vi "(17) part 2 que.vi"() -> ()   [LabVIEW 2025]
panel:
  out "Numeric 2":dbl
  in  "Numeric":dbl
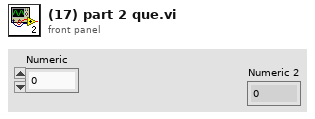
[diagram p1: front panel]
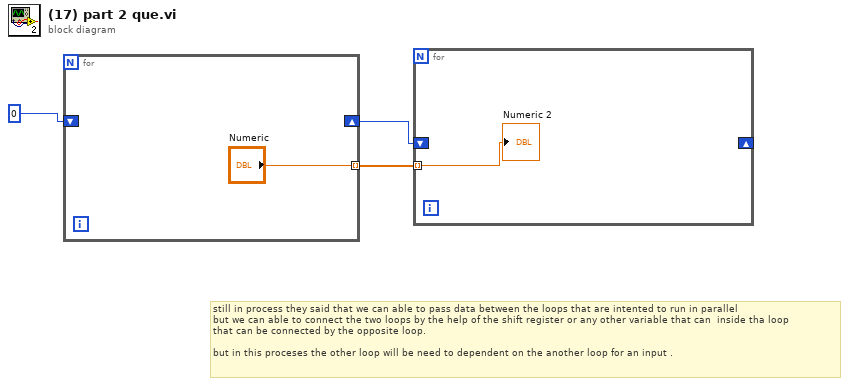
[diagram p0: block diagram]
diagram:
  # "still in process they said that we can able to pass data between the loops that are intented to run in parallel \nbut we can able to connect the two loops by the help of the shift register or any other variable that can  inside tha loop \nthat can be connected by the opposite loop. \n\nbut in this proceses the other loop will be need to dependent on the another loop for an input ."
  n1 = for {
    shift-right: [_] -> w1
    shift-left: 0 -> [_]
    tunnel: ["Numeric"] -> w2 mode=indexing
  }
  n2 = for {
    shift-right: _ -> [_]
    shift-left: w1 -> [_]
    tunnel: w2 -> [w5] mode=indexing
    "Numeric 2" <- w5
  }
